vi "Default Instrument Setup.vi"(8 "error in":errorcluster, 11 "VISA resource name":refnum<visa-resource-name>) -> (0 "error out":errorcluster, 3 "VISA resource name out":refnum<visa-resource-name>)   [LabVIEW 2015, in "IT-M3400.lvlib"]
doc: "Sends a default command string to the instrument whenever a new VISA session is opened, or the instrument is reset. Use this VI as a subVI for the <b>Initialize</b> and <b>Reset</b> VIs. Altering this VI could cause these two VIs to operate incorrectly."
uses:
  <instrlib>/IT-M3400/IT-M3400.lvlib
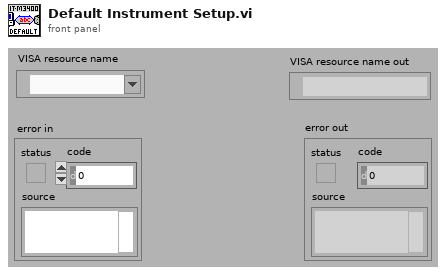
[diagram p1: front panel]
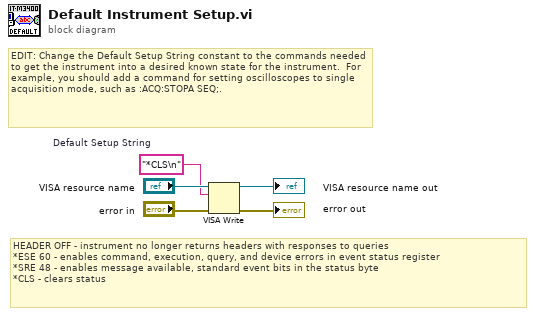
[diagram p0: block diagram]
diagram:
  w1 = "*CLS\n"  # Default Setup String
  # "HEADER OFF - instrument no longer returns headers with responses to queries\n*ESE 60 - enables command, execution, query, and device errors in event status register\n*SRE 48 - enables message available, standard event bits in the status byte\n*CLS - clears status"
  # "EDIT: Change the Default Setup String constant to the commands needed to get the instrument into a desired known state for the instrument.  For example, you should add a command for setting oscilloscopes to single acquisition mode, such as :ACQ:STOPA SEQ;."
  n1 = VISA Write(VISA resource name="VISA resource name", write buffer=w1, error in (no error)="error in") -> (VISA resource name out=→"VISA resource name out":refnum<visa-resource-name>, error out=→"error out":errorcluster)  [unwired: 1 out]
